vi "Get Audio File Tags (UTF-8).vi"(8 "error in (no error)":errorcluster, 11 "Path In":string) -> (0 "error out":errorcluster, 2 "Tags":string[](array[string]), 3 "Path Out":string)   [LabVIEW 2020, in "G-Audio.lvlib"]
doc: "Retrieve audio file tag data.\n\nSupported tag types:\nmp3 (id3v2, id3v1)\nflac (Vorbis comments)"
uses:
  G-Audio.lvlib
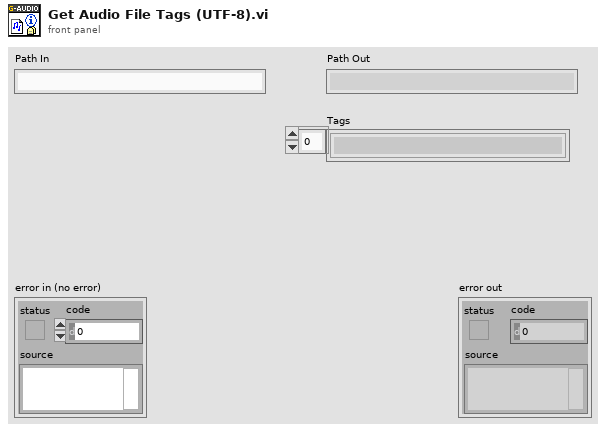
[diagram p1: front panel]
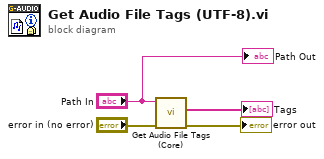
[diagram p0: block diagram]
diagram:
  n1 = call "Get Audio File Tags (Core).vi"("error in (no error)"="error in (no error)", "Path In"="Path In") -> ("error out"=→"error out":errorcluster, "Tags"=→"Tags":string[])  [unwired: 7 in, 1 out]
  "Path Out" <- "Path In"
